vi "Temp_Hum_Calibration.vi"() -> ()   [LabVIEW 2012]
panel:
  out "Outside hum. offset":i32
  out "Outside temp. offset":dbl
  out "Inside hum. offset":i32
  out "Inside temp offset":dbl
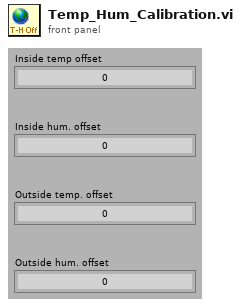
[diagram p1: front panel]
diagram:
